vi "Step Counter.End Subsection.vi"(1 "Step State":T1) -> (0 "Step State Out":T1)   [LabVIEW 2018]
uses:
  Step Counter.State Info.ctl
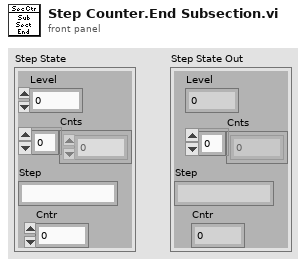
[diagram p1: front panel]
types:
  T1 = typedef "Step Counter.State Info.ctl" = cluster{"Level":i32, "Cnts":i32[], "Step":string, "Cntr":i32}
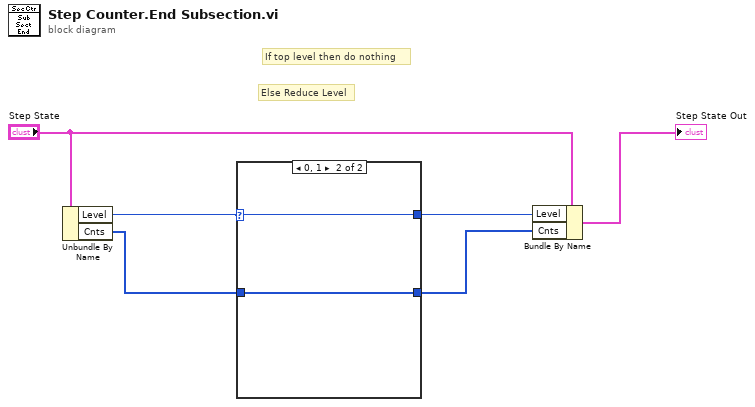
[diagram p0: block diagram]
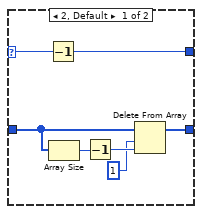
[diagram p2: hidden frame]
diagram:
  # "Else Reduce Level"
  # "If top level then do nothing"
  n1 = Unbundle By Name("Step State") -> ("Level"=w4:i32, "Cnts"=w6:i32[])
  n2 = case shown="0, 1" w4 {
    selector: w4 -> [w8 w14]
    tunnel: w6 -> [w13 w15]
    tunnel: [w9 w15] -> w5
    tunnel: [w7 w14] -> w3
    frame 2, Default {
      n3 = Decrement(x=w8) -> (x-1=w7:i32)
      n4 = Array Size(array=w13) -> (size(s)=w12:i32)
      n5 = Decrement(x=w12) -> (x-1=w11:i32)
      n6 = Delete From Array(array=w13, length=1, index=w11) -> (array with subset deleted=w9:i32[])  [unwired: 1 out]
    }
    frame 0, 1 {
    }
  }
  n7 = Bundle By Name(cluster="Step State", "Level"=w3, "Cnts"=w5) -> (→"Step State Out":T1)
